vi "Update Custom Device XML.vi"(7 "Build Spec Type":string, 8 "error in (no error)":errorcluster, 10 "CD XML/Project Path":path, 11 "Packed Library Path":path) -> (0 "error out":errorcluster, 2 "Project XML Editor out":refnum<class "Project XML Editor.lvclass">)   [LabVIEW 2019, in "LVLIBP CD XML Updater.lvlib"]
uses:
  LVLIBP CD XML Updater.lvlib
  Project XML Editor/Project XML Editor.lvclass
  LVLIBP Parser/LVLIBP Parser.lvclass/LVLIBP Parser.ctl
  Project XML Editor/Project XML Editor.lvclass/Project XML Editor.ctl
  <vilib>/xml/Close Reference(Node).vi
  LVLIBP Parser/LVLIBP Parser.lvclass
  <vilib>/xml/NI_XML.lvlib
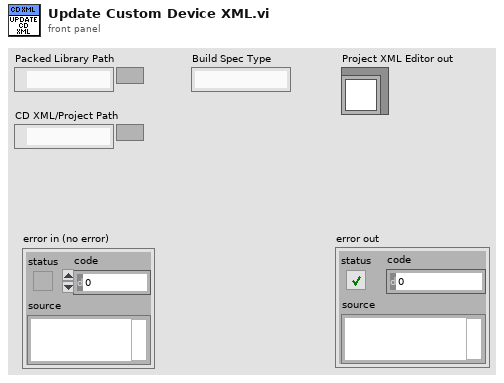
[diagram p1: front panel]
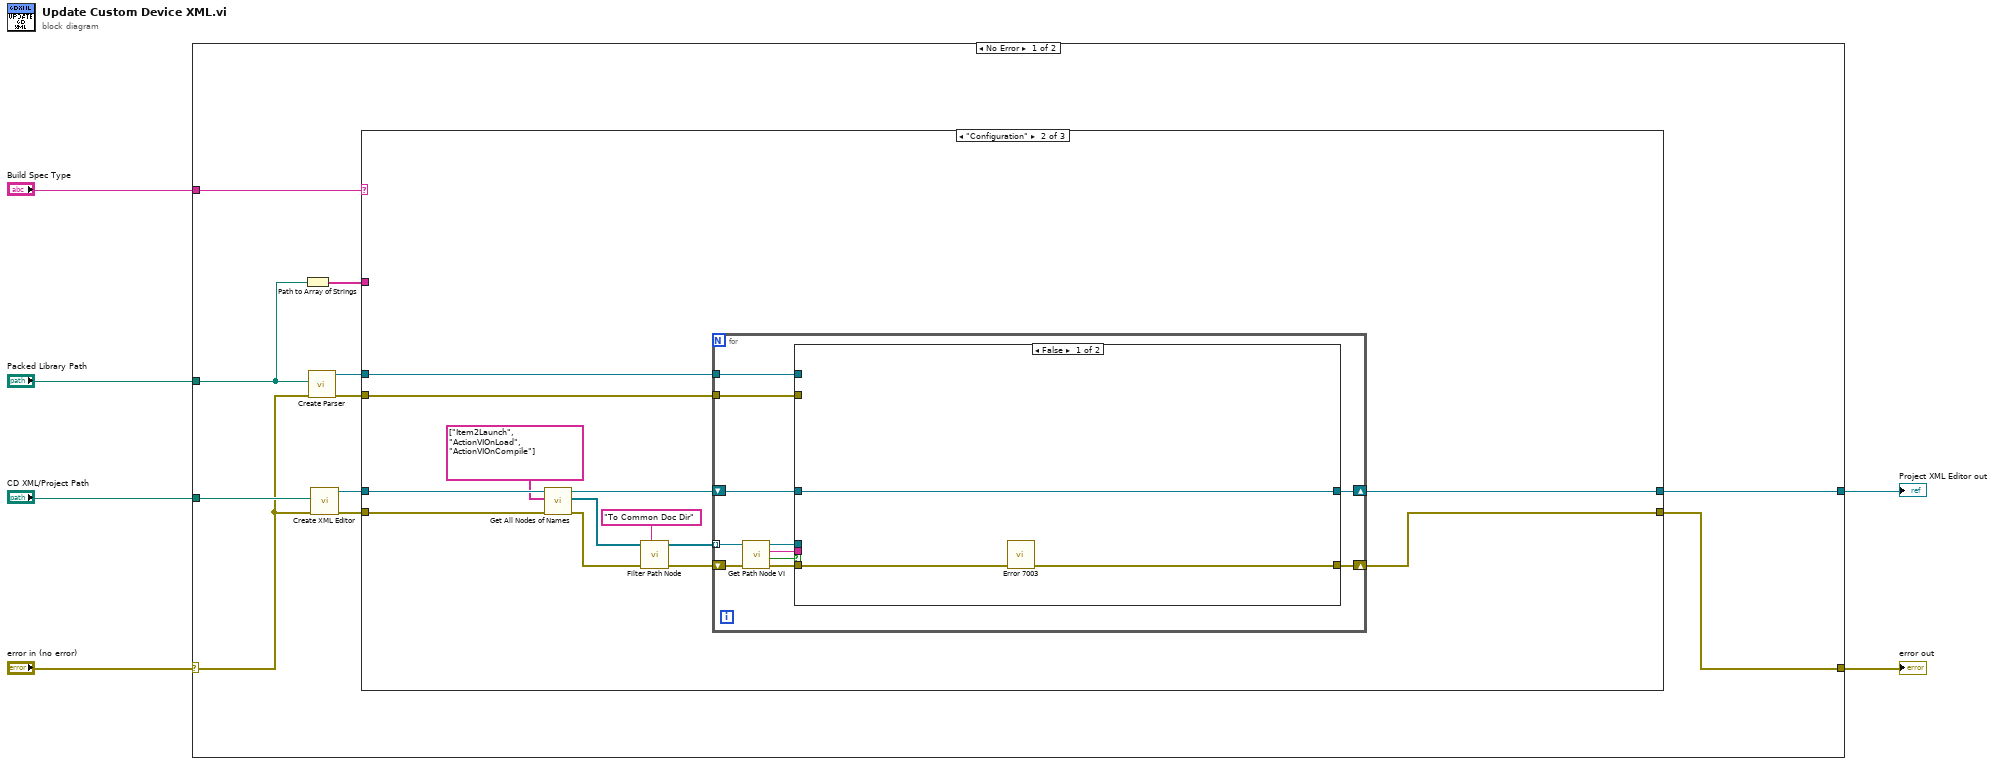
[diagram p0: block diagram]
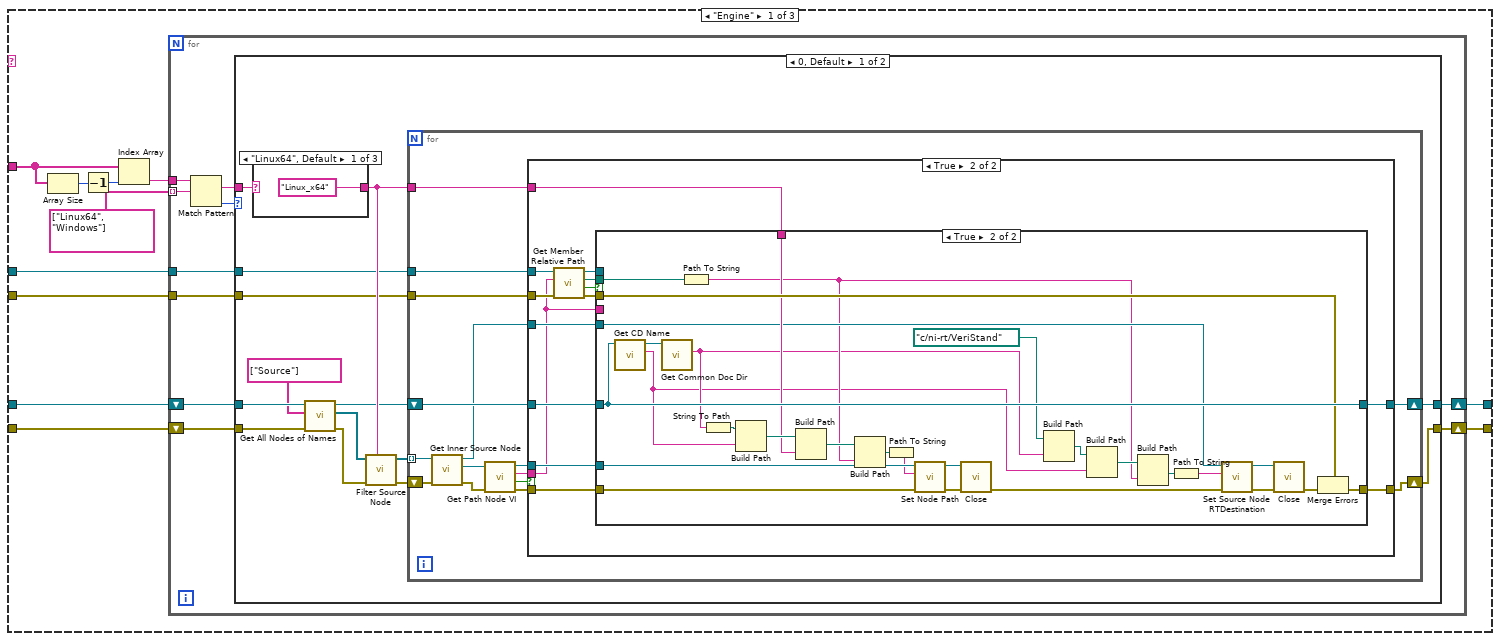
[diagram p2: hidden frame]
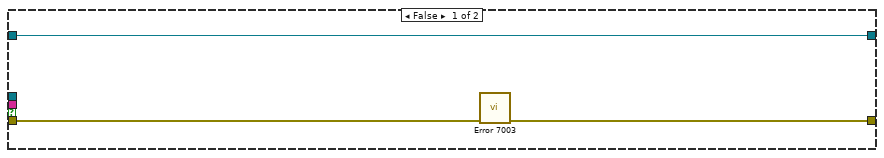
[diagram p3: hidden frame]
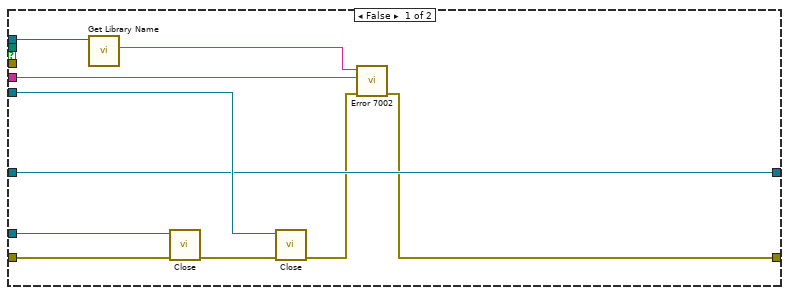
[diagram p4: hidden frame]
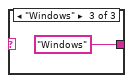
[diagram p6: hidden frame]
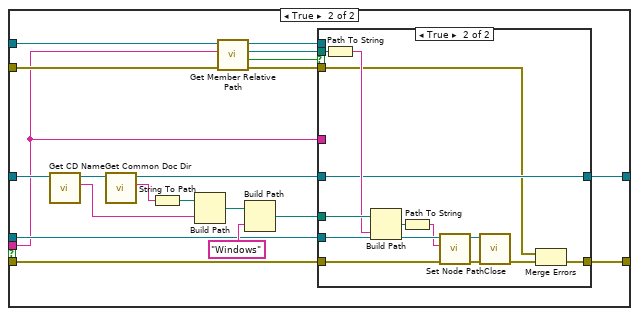
[diagram p8: hidden frame]
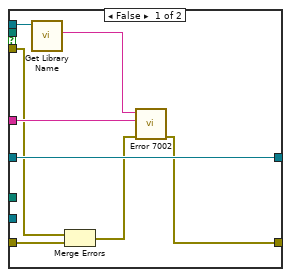
[diagram p9: hidden frame]
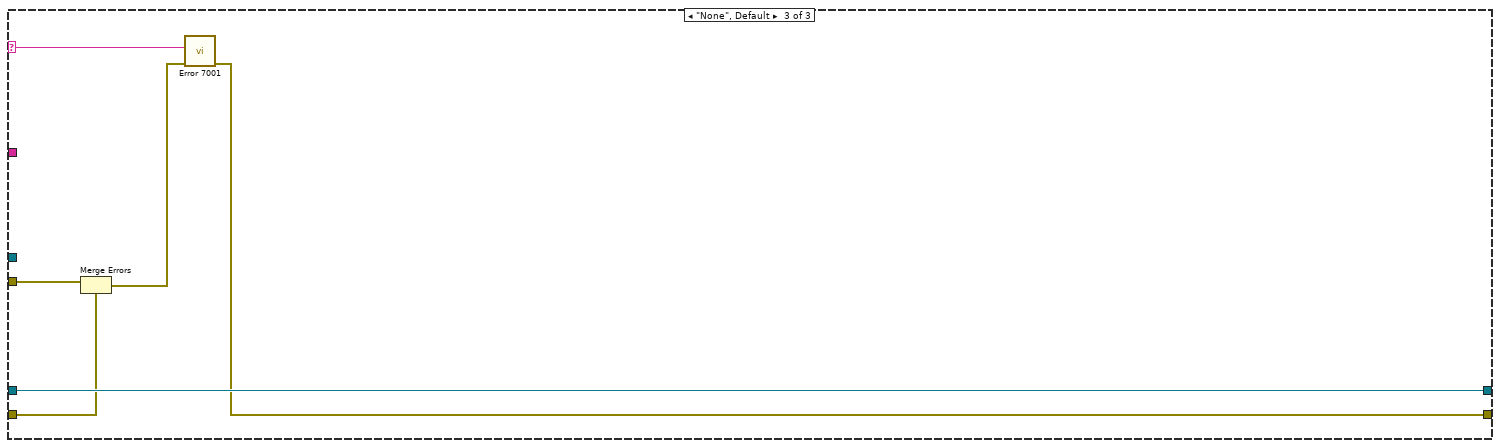
[diagram p10: hidden frame]
diagram:
  n1 = case shown="No Error" "error in (no error)" {
    selector: "error in (no error)" -> [w7 w200]
    tunnel: "Packed Library Path" -> [w16 _]
    tunnel: [w15 _] -> w5
    tunnel: [w14 w200] -> w4
    tunnel: "Build Spec Type" -> [w13 _]
    tunnel: "CD XML/Project Path" -> [w12 _]
    frame No Error {
      n2 = Path to Array of Strings(0:w16) -> (2:w17:string[])  [unwired: 1 out]
      n3 = call "Create Parser.vi"("error in (no error)"=w7, "LVLIBP Path"=w16) -> ("error out"=w9:errorcluster, "LVLIBP Parser out"=w8:refnum<class "LVLIBP Parser.lvclass">)  [unwired: 8 in]
      n4 = call "Create XML Editor.vi"("error in (no error)"=w7, "XML or Project Path"=w12) -> ("error out"=w10:errorcluster, "Project XML Editor out"=w11:refnum<class "Project XML Editor.lvclass">)  [unwired: 8 in]
      n5 = case shown="\"Configuration\"" w13 {
        selector: w13 -> [_ _ w198]
        tunnel: w8 -> [w25 w129 _]
        tunnel: w9 -> [w24 w128 w196]
        tunnel: w10 -> [w28 w136 w195]
        tunnel: w11 -> [w27 w138 w199]
        tunnel: [w22 w130 w197] -> w14
        tunnel: [w23 w126 w199] -> w15
        tunnel: w17 -> [w21 _ _]
        frame "Engine" {
          n6 = Array Size(array=w21) -> (size(s)=w20:i32)
          n7 = Decrement(x=w20) -> (x-1=w19:i32)
          n8 = Index Array(array=w21, index=w19) -> (element=w18:string)
          n9 = for {
            tunnel: string[] ["Linux64", "Windows"] ("Node Names") -> [w36] mode=indexing
            tunnel: w25 -> [w33]
            tunnel: w24 -> [w32]
            shift-right: [w31] -> w23
            shift-left: w27 -> [w37]
            shift-right: [w30] -> w22
            shift-left: w28 -> [w38]
            tunnel: w18 -> [w29]
            n10 = Match Pattern(string=w29, regular expression=w36) -> (match substring=w34:string, offset past match=w35:i32)  [unwired: 1 in, 2 out]
            n11 = case shown="0, Default" w35 {
              tunnel: w38 -> [w52 w124]
              tunnel: w37 -> [w51 w125]
              tunnel: w34 -> [w47 _]
              tunnel: w33 -> [w43 _]
              tunnel: w32 -> [w42 _]
              tunnel: [w40 w125] -> w31
              tunnel: [w39 w124] -> w30
              frame 0, Default {
                n12 = case shown="\"Linux64\", Default" w47 {
                  tunnel: ["Linux_x64" _ "Windows"] -> w44
                  frame "Linux64", Default {
                  }
                  frame "None" {
                  }
                  frame "Windows" {
                  }
                }
                n13 = call "Get All Nodes of Names.vi"("error in (no error)"=w52, "Node Names"=string[] ["Source"], "Project XML Editor in"=w51) -> ("error out"=w48:errorcluster, "Nodes Array out"=w49:refnum<k20>[], "Project XML Editor out"=w41:refnum<class "Project XML Editor.lvclass">)  [unwired: 6 in]
                n14 = call "Filter Source Node.vi"("Supported Target Type"=w44, "error in"=w48, "Nodes Array in"=w49) -> ("error out"=w45:errorcluster, "Nodes Array out"=w46:refnum<k20>[])  [unwired: 7 in]
                n15 = for {
                  tunnel: w46 -> [w66] mode=indexing
                  tunnel: w44 -> [w56]
                  tunnel: w43 -> [w58]
                  tunnel: w42 -> [w57]
                  shift-right: [w55] -> w40
                  shift-left: w41 -> [w59]
                  shift-right: [w54] -> w39
                  shift-left: w45 -> [w67]
                  n16 = call "Get Inner Source Node.vi"("error in (no error)"=w67, "Node ref in"=w66) -> ("error out"=w64:errorcluster, "Inner Source Node"=w65:refnum<k20>, "Node ref out"=w53:refnum<k20>)  [unwired: 6 in, 1 out]
                  n17 = call "Get Path Node VI.vi"("error in (no error)"=w64, "Node ref in"=w65) -> ("error out"=w63:errorcluster, "Found ?"=w62:bool, "VI Name out"=w61:string, "Node ref out"=w60:refnum<k20>)  [unwired: 6 in]
                  n18 = case shown="True" w62 {
                    tunnel: w61 -> [_ w71]
                    tunnel: w59 -> [w70 w74]
                    tunnel: w60 -> [_ w82]
                    tunnel: w63 -> [w69 w81]
                    tunnel: [w68 w79] -> w54
                    tunnel: [w70 w74] -> w55
                    tunnel: w58 -> [_ w78]
                    tunnel: w57 -> [_ w77]
                    tunnel: w56 -> [_ w76]
                    tunnel: w53 -> [_ w75]
                    frame False {
                      n19 = call "Error 7003.vi"("error in (no error)"=w69) -> ("error out"=w68:errorcluster)  [unwired: 10 in]
                    }
                    frame True {
                      n20 = call "Get Member Relative Path.vi"("error in (no error)"=w77, "Member Name"=w71, "LVLIBP Parser in"=w78) -> ("error out"=w80:errorcluster, "Found ?"=w73:bool, "Path"=w83:path, "LVLIBP Parser out"=w72:refnum<class "LVLIBP Parser.lvclass">)  [unwired: 5 in]
                      n21 = case shown="True" w73 {
                        tunnel: w83 -> [_ w119]
                        tunnel: w82 -> [w93 w117]
                        tunnel: w81 -> [w92 w116]
                        tunnel: w80 -> [_ w114]
                        tunnel: [w84 w113] -> w79
                        tunnel: w76 -> [_ w112]
                        tunnel: w75 -> [w91 w111]
                        tunnel: w74 -> [w89 w94]
                        tunnel: [w89 w94] -> _
                        tunnel: w72 -> [w86 _]
                        tunnel: w71 -> [w87 _]
                        frame False {
                          n22 = call "Get Library Name.vi"("LVLIBP Parser in"=w86) -> ("Library Name"=w85:string)  [unwired: 9 in, 1 out]
                          n23 = call-poly <vilib>:"Close.vi"("error in (no error)"=w92, "node"=w93) -> ("error out"=w90:errorcluster)  [unwired: 7 in]
                          n24 = call-poly <vilib>:"Close.vi"("error in (no error)"=w90, "node"=w91) -> ("error out"=w88:errorcluster)  [unwired: 7 in]
                          n25 = call "Error 7002.vi"("error in (no error)"=w88, "VI name in"=w87, "Packekd library name in"=w85) -> ("error out"=w84:errorcluster)  [unwired: 8 in]
                        }
                        frame True {
                          n26 = call "Get CD Name.vi"("Project XML Editor in"=w94) -> ("CD Name"=w99:string, "Project XML Editor out"=w115:refnum<class "Project XML Editor.lvclass">)  [unwired: 9 in]
                          n27 = call "Get Common Doc Dir.vi"("Project XML Editor in"=w115) -> ("Common Doc Dir"=w100:string)  [unwired: 9 in, 1 out]
                          n28 = Path To String(path=w119) -> (string=w102:string)
                          n29 = String To Path(string=w100) -> (path=w121:path)
                          n30 = Build Path(base path=w121, name or relative path=w99) -> (appended path=w120:path)
                          n31 = Build Path(base path=w120, name or relative path=w112) -> (appended path=w118:path)
                          n32 = Build Path(base path=w118, name or relative path=w102) -> (appended path=w106:path)
                          n33 = Path To String(path=w106) -> (string=w105:string)
                          n34 = call "Set Node Path.vi"("error in (no error)"=w116, "Path in"=w105, "Node ref in"=w117) -> ("error out"=w104:errorcluster, "Node ref out"=w103:refnum<k20>)  [unwired: 6 in, 1 out]
                          n35 = call-poly <vilib>:"Close.vi"("error in (no error)"=w104, "node"=w103) -> ("error out"=w110:errorcluster)  [unwired: 7 in]
                          n36 = Build Path(base path=path "c:/ni-rt/VeriStand", name or relative path=w100) -> (appended path=w108:path)
                          n37 = Build Path(base path=w108, name or relative path=w99) -> (appended path=w107:path)
                          n38 = Build Path(base path=w107, name or relative path=w102) -> (appended path=w101:path)
                          n39 = Path To String(path=w101) -> (string=w98:string)
                          n40 = call "Set Source Node RTDestination.vi"("error in (no error)"=w110, "Path in"=w98, "Node ref in"=w111) -> ("error out"=w97:errorcluster, "Node ref out"=w96:refnum<k20>)  [unwired: 6 in, 1 out]
                          n41 = call-poly <vilib>:"Close.vi"("error in (no error)"=w97, "node"=w96) -> ("error out"=w95:errorcluster)  [unwired: 7 in]
                          n42 = Merge Errors(w114, w95) -> (w113:errorcluster)
                        }
                      }
                    }
                  }
                }
              }
              frame -1 {
              }
            }
          }
        }
        frame "Configuration" {
          n43 = call "Get All Nodes of Names.vi"("error in (no error)"=w136, "Node Names"=string[] ["Item2Launch", "ActionVIOnLoad", "ActionVIOnCompile"], "Project XML Editor in"=w138) -> ("error out"=w135:errorcluster, "Nodes Array out"=w134:refnum<k20>[], "Project XML Editor out"=w127:refnum<class "Project XML Editor.lvclass">)  [unwired: 6 in]
          n44 = call "Filter Path Node.vi"("Node Path Type"="To Common Doc Dir" ("y"), "error in"=w135, "Nodes Array in"=w134) -> ("error out"=w131:errorcluster, "Nodes Array out"=w132:refnum<k20>[])  [unwired: 7 in]
          n45 = for {
            tunnel: w132 -> [w149] mode=indexing
            shift-right: [w142] -> w130
            shift-left: w131 -> [w148]
            tunnel: w128 -> [w139]
            shift-right: [w140] -> w126
            shift-left: w127 -> [w145]
            tunnel: w129 -> [w147]
            n46 = call "Get Path Node VI.vi"("error in (no error)"=w148, "Node ref in"=w149) -> ("error out"=w143:errorcluster, "Found ?"=w141:bool, "VI Name out"=w146:string, "Node ref out"=w144:refnum<k20>)  [unwired: 6 in]
            n47 = case shown="False" w141 {
              tunnel: w147 -> [_ w172]
              tunnel: w146 -> [_ w156]
              tunnel: w145 -> [w152 w162]
              tunnel: w144 -> [_ w164]
              tunnel: w143 -> [w151 w163]
              tunnel: [w150 w153] -> w142
              tunnel: [w152 w157] -> w140
              tunnel: w139 -> [_ w159]
              frame False {
                n48 = call "Error 7003.vi"("error in (no error)"=w151) -> ("error out"=w150:errorcluster)  [unwired: 10 in]
              }
              frame True {
                n49 = call "Get CD Name.vi"("Project XML Editor in"=w162) -> ("CD Name"=w160:string, "Project XML Editor out"=w161:refnum<class "Project XML Editor.lvclass">)  [unwired: 9 in]
                n50 = call "Get Common Doc Dir.vi"("Project XML Editor in"=w161) -> ("Common Doc Dir"=w171:string, "Project XML Editor out"=w158:refnum<class "Project XML Editor.lvclass">)  [unwired: 9 in]
                n51 = String To Path(string=w171) -> (path=w170:path)
                n52 = Build Path(base path=w170, name or relative path=w160) -> (appended path=w169:path)
                n53 = call "Get Member Relative Path.vi"("error in (no error)"=w159, "Member Name"=w156, "LVLIBP Parser in"=w172) -> ("error out"=w154:errorcluster, "Found ?"=w167:bool, "Path"=w166:path, "LVLIBP Parser out"=w155:refnum<class "LVLIBP Parser.lvclass">)  [unwired: 5 in]
                n54 = Build Path(base path=w169, name or relative path="Windows") -> (appended path=w165:path)
                n55 = case shown="True" w167 {
                  tunnel: w166 -> [_ w193]
                  tunnel: w165 -> [_ w192]
                  tunnel: w164 -> [_ w190]
                  tunnel: w163 -> [w175 w187]
                  tunnel: [w173 w181] -> w153
                  tunnel: w158 -> [w180 w186]
                  tunnel: [w180 w186] -> w157
                  tunnel: w156 -> [w179 _]
                  tunnel: w155 -> [w178 _]
                  tunnel: w154 -> [w176 w182]
                  frame False {
                    n56 = call "Get Library Name.vi"("LVLIBP Parser in"=w178) -> ("Library Name"=w177:string)  [unwired: 9 in, 1 out]
                    n57 = Merge Errors(w176, w175) -> (w174:errorcluster)
                    n58 = call "Error 7002.vi"("error in (no error)"=w174, "VI name in"=w179, "Packekd library name in"=w177) -> ("error out"=w173:errorcluster)  [unwired: 8 in]
                  }
                  frame True {
                    n59 = Path To String(path=w193) -> (string=w191:string)
                    n60 = Build Path(base path=w192, name or relative path=w191) -> (appended path=w189:path)
                    n61 = Path To String(path=w189) -> (string=w188:string)
                    n62 = call "Set Node Path.vi"("error in (no error)"=w187, "Path in"=w188, "Node ref in"=w190) -> ("error out"=w185:errorcluster, "Node ref out"=w184:refnum<k20>)  [unwired: 6 in, 1 out]
                    n63 = call-poly <vilib>:"Close.vi"("error in (no error)"=w185, "node"=w184) -> ("error out"=w183:errorcluster)  [unwired: 7 in]
                    n64 = Merge Errors(w182, w183) -> (w181:errorcluster)
                  }
                }
              }
            }
          }
        }
        frame "None", Default {
          n65 = Merge Errors(w196, w195) -> (w194:errorcluster)
          n66 = call "Error 7001.vi"("error in (no error)"=w194, "Build type in"=w198) -> ("error out"=w197:errorcluster)  [unwired: 9 in]
        }
      }
    }
    frame Error {
    }
  }
  "Project XML Editor out" <- w5
  "error out" <- w4
